vi "Instantiate Sink.vi"(11 "Log Sink in":refnum<class "Log Sink.lvclass">) -> (0 "error out":errorcluster, 3 "Log Sink Reference":refnum<data-value>)   [LabVIEW 2019, in "Composed Log.lvlib" / "Log Sink.lvclass"]
uses:
  <vilib>/gpm_packages/@cs/event-logger/Source/Composed Log/Log Sink/Log Sink.lvclass
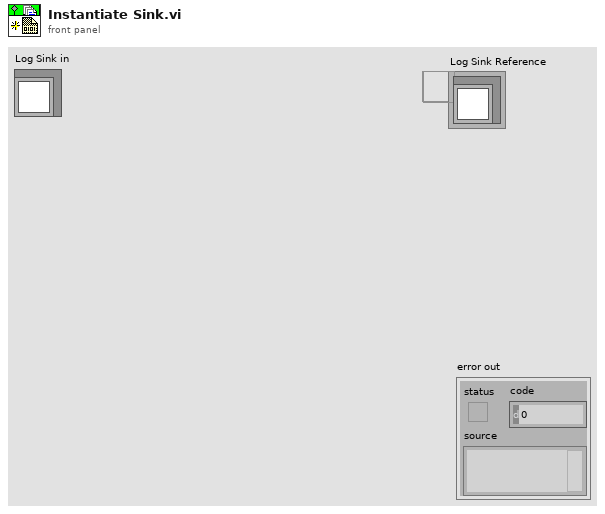
[diagram p1: front panel]
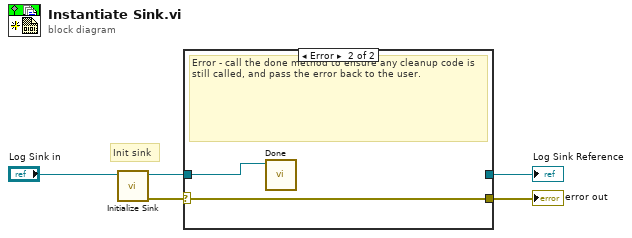
[diagram p0: block diagram]
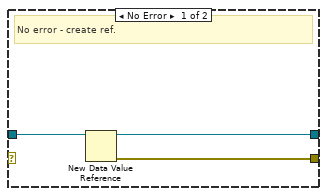
[diagram p2: hidden frame]
diagram:
  # "Init sink"
  n1 = call-dynamic "Initialize Sink.vi"("Log Sink in"="Log Sink in") -> ("error out"=w3:errorcluster, "Log Sink out"=w4:refnum<class "Log Sink.lvclass">)  [unwired: 9 in]
  n2 = case shown="Error" w3 {
    selector: w3 -> [_ w10]
    tunnel: w4 -> [w8 w9]
    tunnel: [w7 _] -> w1
    tunnel: [w6 w10] -> w2
    frame No Error {
      # "No error - create ref."
      n3 = New Data Value Reference(data value=w8) -> (data value reference=w7:refnum<data-value>, error out=w6:errorcluster)  [unwired: 1 in]
    }
    frame Error {
      # "Error - call the done method to ensure any cleanup code is still called, and pass the error back to the user."
      n4 = call-dynamic "Done.vi"("Log Sink in"=w9) -> ()  [unwired: 10 in, 1 out]
    }
  }
  "error out" <- w2
  "Log Sink Reference" <- w1
